vi "A-Weight (given frequency).vi"(2 "Frequency (Hz)":dbl=1.0) -> (16 "A-Weight (dB)":dbl)   [LabVIEW 2020, in "GSwFormDSP.lvclass"]
uses:
  GSwFormDSP.lvclass
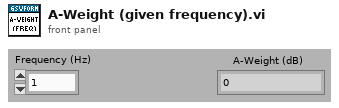
[diagram p1: front panel]
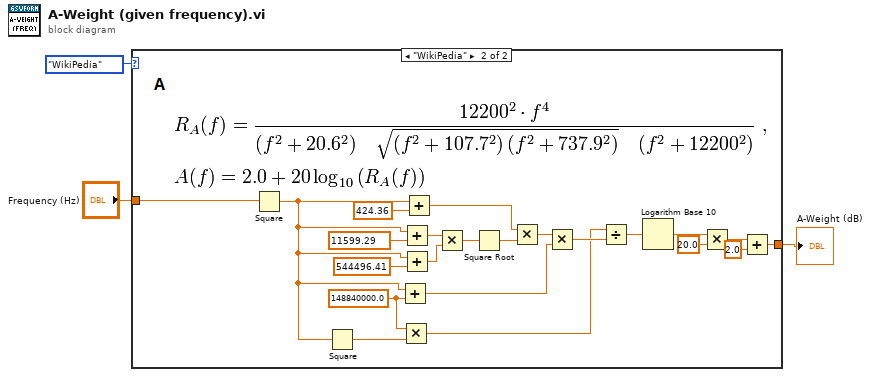
[diagram p0: block diagram]
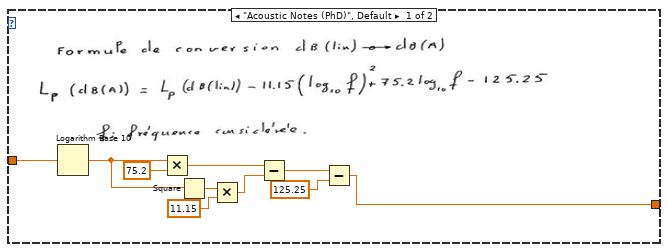
[diagram p2: hidden frame]
diagram:
  n1 = case shown="\"WikiPedia\"" enum16{"Acoustic Notes (PhD)", "WikiPedia"}."WikiPedia" ("Equation Source") {
    tunnel: [w4 w35] -> w3
    tunnel: "Frequency (Hz)" -> [w13 w14]
    frame "Acoustic Notes (PhD)", Default {
      n2 = Logarithm Base 10(1:w13) -> (0:w11:dbl)
      n3 = Multiply(x=w11, y=75.2) -> (x*y=w8:dbl)
      n4 = Square(x=w11) -> (x^2=w10:dbl)
      n5 = Multiply(x=w10, y=11.15) -> (x*y=w7:dbl)
      n6 = Subtract(x=w8, y=w7) -> (x-y=w6:dbl)
      n7 = Subtract(x=w6, y=125.25) -> (x-y=w4:dbl)
    }
    frame "WikiPedia" {
      w25 = 148840000.0 ("y")
      n8 = Square(x=w14) -> (x^2=w26:dbl)
      n9 = Square(x=w26) -> (x^2=w27:dbl)
      n10 = Add(x=w26, y=w25) -> (x+y=w24:dbl)
      n11 = Multiply(x=w25, y=w27) -> (x*y=w28:dbl)
      n12 = Add(x=w26, y=11599.29) -> (x+y=w18:dbl)
      n13 = Add(x=w26, y=544496.41) -> (x+y=w19:dbl)
      n14 = Add(x=w26, y=424.36) -> (x+y=w22:dbl)
      n15 = Multiply(x=w18, y=w19) -> (x*y=w20:dbl)
      n16 = Square Root(x=w20) -> (sqrt(x)=w21:dbl)
      n17 = Multiply(x=w22, y=w21) -> (x*y=w23:dbl)
      n18 = Multiply(x=w23, y=w24) -> (x*y=w29:dbl)
      n19 = Divide(x=w28, y=w29) -> (x/y=w30:dbl)
      n20 = Logarithm Base 10(1:w30) -> (0:w31:dbl)
      n21 = Multiply(x=w31, y=20.0) -> (x*y=w33:dbl)
      n22 = Add(x=w33, y=2.0) -> (x+y=w35:dbl)
    }
  }
  "A-Weight (dB)" <- w3
